vi "Generate_Consumer_study(1).vi"() -> ()   [LabVIEW 2017]
panel:
  out "웰치스 2":bool
  out "콜라 2":bool
  out "환타 2":bool
  out "사이다 2":bool
  out "배달 상품명":string
  out "현재잔액":dbl
  in  "클러스터":T1
  in  "사이다":bool
  in  "콜라":bool
  in  "환타":bool
  in  "웰치스":bool
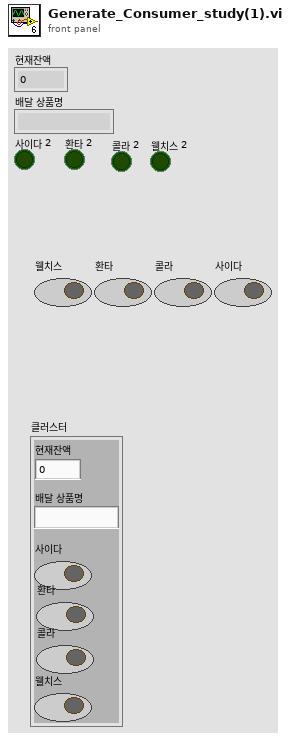
[diagram p1: front panel]
types:
  T1 = cluster{"현재잔액":dbl, "배달 상품명":string, "사이다":bool, "환타":bool, "콜라":bool, "웰치스":bool}
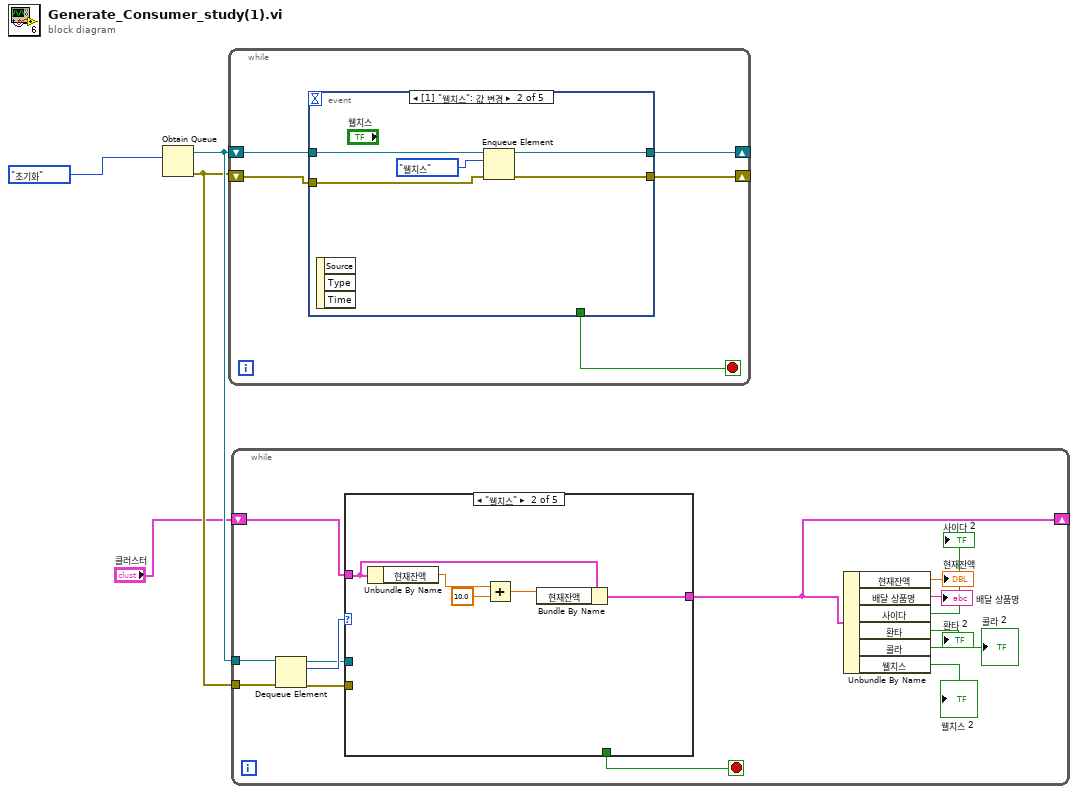
[diagram p0: block diagram]
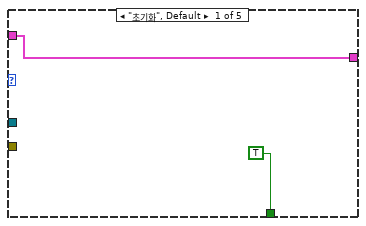
[diagram p2: hidden frame]
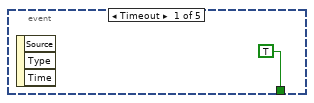
[diagram p6: hidden frame]
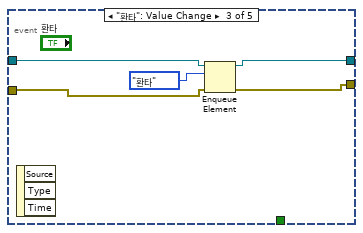
[diagram p7: hidden frame]
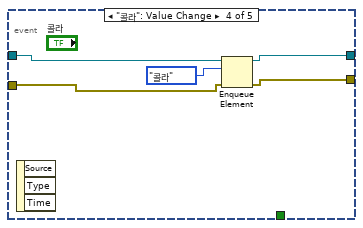
[diagram p8: hidden frame]
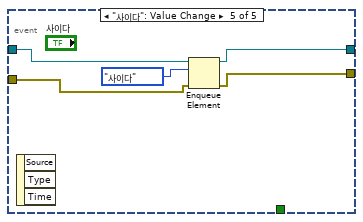
[diagram p9: hidden frame]
diagram:
  n1 = Obtain Queue(element data type=enum16{"초기화", "웰치스", "사이다", "환타", "콜라"}."초기화" ("열거형")) -> (queue out=w3:refnum<queue>, error out=w2:errorcluster)  [unwired: 4 in, 1 out]
  n2 = while {
    shift-right: [w5] -> _
    shift-left: w3 -> [w8]
    shift-right: [w6] -> _
    shift-left: w2 -> [w7]
    stop <- w9 stop-if-true
    n3 = event shown="[1] \"웰치스\": 값 변경" {
      selector: _ -> [_ _ _ _ _]
      dyn-events: _ -> [_ _ _ _ _]
      timeout: _ -> [_ _ _ _ _]
      tunnel: [TRUE _ _ _ _] -> w9
      tunnel: w8 -> [_ w15 w19 w24 w29]
      tunnel: w7 -> [_ w13 w16 w22 w27]
      tunnel: [_ w12 w17 w21 w26] -> w6
      tunnel: [_ w11 w18 w23 w28] -> w5
      event Timeout {
        n4 = event-data() -> ()  [unwired: 1 in, 3 out]
      }
      event "웰치스": Value Change {
        n5 = event-data() -> ()  [unwired: 1 in, 3 out]
        n6 = Enqueue Element(queue=w15, element=enum16{"초기화", "웰치스", "사이다", "환타", "콜라"}."웰치스" ("열거형"), error in (no error)=w13) -> (queue out=w11:refnum<queue>, error out=w12:errorcluster)  [unwired: 1 in, 1 out]
      }
      event "환타": Value Change {
        n7 = event-data() -> ()  [unwired: 1 in, 3 out]
        n8 = Enqueue Element(queue=w19, element=enum16{"초기화", "웰치스", "사이다", "환타", "콜라"}."환타" ("열거형"), error in (no error)=w16) -> (queue out=w18:refnum<queue>, error out=w17:errorcluster)  [unwired: 1 in, 1 out]
      }
      event "콜라": Value Change {
        n9 = event-data() -> ()  [unwired: 1 in, 3 out]
        n10 = Enqueue Element(queue=w24, element=enum16{"초기화", "웰치스", "사이다", "환타", "콜라"}."콜라" ("열거형"), error in (no error)=w22) -> (queue out=w23:refnum<queue>, error out=w21:errorcluster)  [unwired: 1 in, 1 out]
      }
      event "사이다": Value Change {
        n11 = event-data() -> ()  [unwired: 1 in, 3 out]
        n12 = Enqueue Element(queue=w29, element=enum16{"초기화", "웰치스", "사이다", "환타", "콜라"}."사이다" ("열거형"), error in (no error)=w27) -> (queue out=w28:refnum<queue>, error out=w26:errorcluster)  [unwired: 1 in, 1 out]
      }
    }
  }
  n13 = while {
    tunnel: w3 -> [w44]
    tunnel: w2 -> [w43]
    shift-right: [w31] -> _
    shift-left: "클러스터" -> [w39]
    stop <- w38 stop-if-true
    n14 = Dequeue Element(queue=w44, error in (no error)=w43) -> (queue out=w41:refnum<queue>, element=w42:enum16{"초기화", "웰치스", "사이다", "환타", "콜라"}, error out=w40:errorcluster)  [unwired: 1 in, 1 out]
    n15 = case shown="\"웰치스\"" w42 {
      tunnel: w41 -> [_ _ _ _ _]
      tunnel: w40 -> [_ _ _ _ _]
      tunnel: w39 -> [w46 w48 _ _ _]
      tunnel: [w46 w47 _ _ _] -> w31
      tunnel: [TRUE _ _ _ _] -> w38
      frame "초기화", Default {
      }
      frame "웰치스" {
        n16 = Unbundle By Name(w48) -> ("현재잔액"=w51:dbl)
        n17 = Add(x=w51, y=10.0) -> (x+y=w49:dbl)
        n18 = Bundle By Name(cluster=w48, "현재잔액"=w49) -> (w47:T1)
      }
      frame "사이다" {
      }
      frame "환타" {
      }
      frame "콜라" {
      }
    }
    n19 = Unbundle By Name(w31) -> ("현재잔액"=→"현재잔액":dbl, "배달 상품명"=→"배달 상품명":string, "사이다"=→"사이다 2":bool, "환타"=→"환타 2":bool, "콜라"=→"콜라 2":bool, "웰치스"=→"웰치스 2":bool)
  }
